vi "Auton Eject Gear.vi"() -> (3 "Done?":bool)   [LabVIEW 2016]
uses:
  <vilib>/Rock Robotics/WPI/Solenoid/WPI_SolenoidValue.ctl
  Robot Values.vi
  Robot Global Reference.vi
  <vilib>/Rock Robotics/WPI/Solenoid/WPI_SolenoidGetEnum.vi
  <vilib>/ptbypt/NI_PtbyPt.lvlib
panel:
  in  "Time to  Wait After Ejection (s)":dbl=1.0 format="%#_13g"
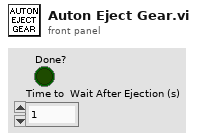
[diagram p1: front panel]
types:
  T1 = typedef "WPI_SolenoidValue.ctl" = enum16{"Off", "On", "Forward", "Reverse"}
  T2 = typedef "Joystick Reference.ctl" = cluster{"Driver Joystick":T3, "Operator Joystick":T3}
  T3 = typedef "WPI_JoystickDevRef.ctl" = cluster{"Device":T4}
  T4 = typedef "WPI_JoystickDeviceEnum.ctl" = enum16{"USB 0", "USB 1", "USB 2", "USB 3", "USB 4", "USB 5"}
  T5 = typedef "Drive Reference.ctl" = cluster{"RobotDriveDevRef":T6, "Drive PTO Solenoid":T11, "High Gear Solenoid":T11}
  T6 = typedef "WPI_RobotDriveDevRef.ctl" = cluster{"DevStatus":errorcluster, "Motors[]":T7[], "Square Inputs":bool, "Max Output":dbl}
  T7 = typedef "WPI_MotorControlDeviceRef.ctl" = cluster{"DeviceStatus":errorcluster, "Type":T8, "PWM":cluster{"PWM Channel":T9, "DeadBand":T10}, "CAN":cluster{"Device Number":u8, "SetOutput VI Ref":variant, "GetOutput VI Ref":variant, "Enable VI Ref":variant, "Disable VI Ref":variant, "Data":variant}, "Invert":bool}
  T8 = typedef "WPI_MotorControlType.ctl" = enum16{"PWM", "CAN"}
  T9 = typedef "FPGA_DIOPWMChannel.ctl" = enum8{"PWM 0", "PWM 1", "PWM 2", "PWM 3", "PWM 4", "PWM 5", "PWM 6", "PWM 7", "PWM 8", "PWM 9", "PWM MXP 0", "PWM MXP 1", "PWM MXP 2", "PWM MXP 3", "PWM MXP 4", "PWM MXP 5", "PWM MXP 6", "PWM MXP 7", "PWM MXP 8", "PWM MXP 9", "Invalid"}
  T10 = typedef "WPI_PWMDeadband.ctl" = cluster{"Name":string, "maxPositivePwm":i32, "minPositivePwm":i32, "centerPwm":i32, "maxNegativePwm":i32, "minNegativePwm":i32, "angularRange":u16}
  T11 = typedef "WPI_SolenoidDevRef.ctl" = cluster{"DevStatus":errorcluster, "Pneumatics Control Module":u8, "Forward Solenoid Channel":T12, "Reverse Solenoid Channel":T12}
  T12 = typedef "WPI_SolenoidChannel.ctl" = enum8{"Solenoid 0", "Solenoid 1", "Solenoid 2", "Solenoid 3", "Solenoid 4", "Solenoid 5", "Solenoid 6", "Solenoid 7", "Invalid"}
  T13 = typedef "Sensor Reference.ctl" = cluster{"LeftMotorEncoderRef":T14, "RightMotorEncoderRef":T14, "I2C Gyro":T18, "Left Shooter Wheel Encoder":T14}
  T14 = typedef "WPI_EncoderDevRef.ctl" = cluster{"DevStatus":errorcluster, "EncoderIndex":T15, "CounterIndex":T16, "DistancePerCount":dbl, "Decoding Type":T17}
  T15 = typedef "FPGA_EncoderIdx.ctl" = enum8{"Enc 0", "Enc 1", "Enc 2", "Enc 3", "Enc 4", "Enc 5", "Enc 6", "Enc 7", "Invalid"}
  T16 = typedef "FPGA_CounterCtrSystemIndex.ctl" = enum8{"Ctr 0", "Ctr 1", "Ctr 2", "Ctr 3", "Ctr 4", "Ctr 5", "Ctr 6", "Ctr 7", "Invalid"}
  T17 = typedef "WPI_EncoderType.ctl" = enum16{"1x", "2x", "4x"}
  T18 = typedef "WPI_I2CDevRef.ctl" = cluster{"DevStatus":errorcluster, "Device Address":u8, "Handle":i32, "I2C Bus":T19}
  T19 = typedef "i2c_bus.ctl" = enum16{"I2C On-Board", "I2C MXP", "Invalid"}
  T20 = typedef "Shoot Reference.ctl" = cluster{"Shooter Wheel Left":T7, "Shooter Wheel Right":T7, "Acquisition Conveyor Motor DevRef":T7, "Hopper Beater Bar Motor DevRef":T7}
  T21 = typedef "Gear Reference.ctl" = cluster{"Gear Ejection Cylinder":T11, "Door Ejection Cylinder":T11}
  T22 = typedef "Light Reference.ctl" = cluster{"SerialPortRef":T23}
  T23 = typedef "WPI_SerialPortRef.ctl" = cluster{"DevStatus":errorcluster, "Serial Port Name":refnum<visa-resource-name>}
  T24 = cluster{"Joystick Reference":T2, "Drive Reference":T5, "Sensor Reference":T13, "Shoot + Aquisition Reference":T20, "Gear Reference":T21, "Acquisition Conveyor Motor DevRef":T7, "Lights":T22}
  T25 = typedef "Robot Values.ctl" = cluster{"Robot Drive":cluster{"Left Motor Power":dbl, "Right Motor Power":dbl, "Left Encoder Value":dbl, "Right Encoder Value":dbl, "High Gear?":bool, "PTO?":bool}, "Sensors":cluster{"Gyro Angle":u16, "Recalibrate Gyro":bool, "Reset Gyro":bool, "Ultrasonic":dbl}, "Shooter":cluster{"Prep Wheels":bool, "Shoot":bool, "Left Shooter Wheel Speed":dbl, "Wheels Moving":bool, "Shooter Prepped":bool, "Shooter RPS SP":dbl, "Shooting?":bool, "Left Shooter Wheel Power":dbl, "Right Shooter Wheel Power":dbl, "Acquisition Conveyor Power":dbl, "Hopper Beater Bar Power":dbl, "Filtered Left Shooter Speed":dbl, "Acquisition Motor Power":dbl, "Joystick Add":dbl}, "Robot States":cluster{"Drive mode":string, "Alliance":T26, "Position":T27}, "Gear":cluster{"Ejection Active":bool}}
  T26 = typedef "WPI_DriverStationAllianceInfo.ctl" = enum16{"Red", "Blue", "Invalid"}
  T27 = typedef "WPI_DriverStationPositionInfo.ctl" = enum16{"1", "2", "3"}
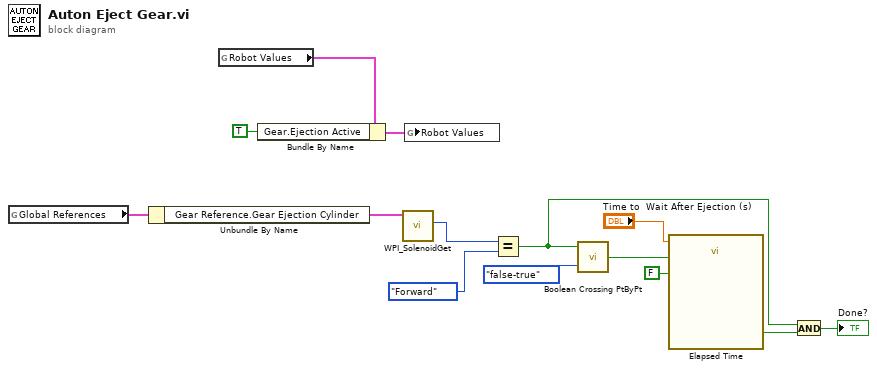
[diagram p0: block diagram]
diagram:
  n1 = global read "Robot Global Reference.vi" "Global References"() -> (w11:T24)
  n2 = Unbundle By Name(w11) -> ("Gear Reference.Gear Ejection Cylinder"=w10:T11)
  n3 = global read "Robot Values.vi" "Robot Values"() -> (w14:T25)
  n4 = Bundle By Name(cluster=w14, "Gear.Ejection Active"=TRUE ("Gear.Ejjection Active")) -> (w13:T25)
  n5 = call-poly <vilib>:"WPI_SolenoidGet.vi"("SolenoidDevRef"=w10) -> ("Value"=w9:T1)  [unwired: 8 in, 2 out]
  n6 = global write "Robot Values.vi" "Robot Values"(w13) -> ()
  n7 = Equal?(x=w9, y=WPI_SolenoidValue."Forward" ("Value")) -> (x = y?=w2:bool)
  n8 = call <vilib>:"Boolean Crossing PtByPt.vi"("direction"=enum16{"either", "false-true", "true-false"}."false-true", "input"=w2) -> ("crossing"=w4:bool)  [unwired: 1 in]
  n9 = call "Elapsed Time"("Time Target (s)"="Time to  Wait After Ejection (s)", "Reset"=w4, "Auto Reset"=FALSE) -> ("Time has Elapsed"=w3:bool)  [unwired: 9 in, 7 out]
  n10 = And(x=w2, y=w3) -> (x .and. y?=→"Done?":bool)
